vi "Stop Instruments.vi"(8 "Error In":errorcluster, 11 "reference in":refnum<class "Measure and Stimulus Subsystems.lvclass">) -> (0 "Error Out":errorcluster, 3 "reference out":refnum<class "Measure and Stimulus Subsystems.lvclass">)   [LabVIEW 2023, in "HAL GOOP4.lvlib" / "Measure and Stimulus Subsystems.lvclass"]
uses:
  Measure and Stimulus Subsystems.lvclass
  Measure and Stimulus Subsystems.lvclass/Measure and Stimulus Subsystems.ctl
  Interfaces/IInstrument/IInstrument.lvclass
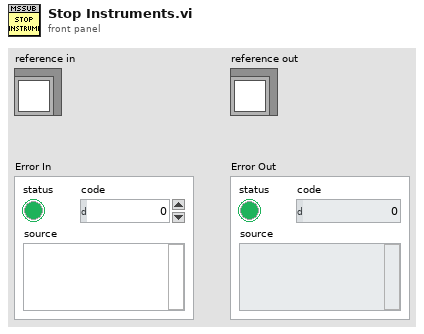
[diagram p1: front panel]
types:
  T1 = typedef "HAL GOOP4.lvlib/Measure and Stimulus Subsystems.lvclass/ObjectAttributes.ctl" = cluster{"Virt Instr":map{string, cluster{"IInstrument Base":refnum<class "IInstrument.lvclass">, "Channel":u8}}, "Physical Instr":map{string, cluster{"IInstrument Base":refnum<class "IInstrument.lvclass">, "Ref Count":u8}}}
  T2 = map{string, cluster{"IInstrument Base":refnum<class "IInstrument.lvclass">, "Ref Count":u8}}
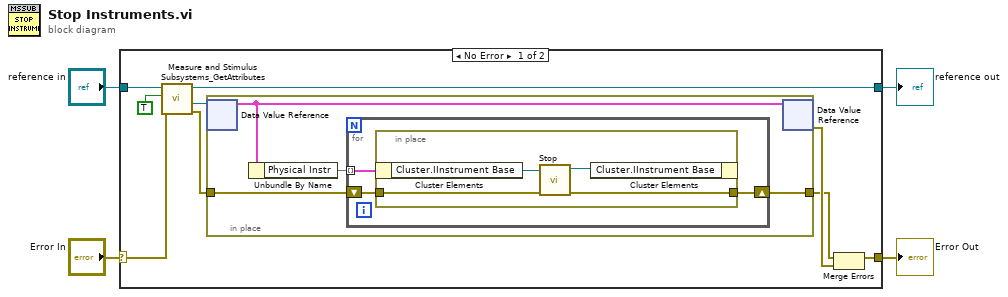
[diagram p0: block diagram]
diagram:
  n1 = case shown="No Error" "Error In" {
    selector: "Error In" -> [w12 w26]
    tunnel: [w9 w26] -> w3
    tunnel: [w10 w25] -> w1
    tunnel: "reference in" -> [w13 w25]
    frame No Error {
      n2 = call "Measure and Stimulus Subsystems_GetAttributes.vi"("Error In"=w12, "OnlyGetDvrReference(False)"=TRUE, "reference in"=w13) -> ("Error Out"=w6:errorcluster, "DataRef"=w8:refnum<data-value>, "reference out"=w10:refnum<class "Measure and Stimulus Subsystems.lvclass">)  [unwired: 5 in, 1 out]
      n3 = in-place {
        in-place-border: [w15] -> w5
        in-place-border: w6 -> [w14]
        n4 = in-place-dvr #1(w8) -> (w16:T1)  [unwired: 1 out]
        n5 = Unbundle By Name(w16) -> ("Physical Instr"=w17:T2)
        n6 = for {
          tunnel: w17 -> [w20] mode=indexing
          shift-right: [w18] -> w15
          shift-left: w14 -> [w19]
          n7 = in-place {
            in-place-border: w19 -> [w22]
            in-place-border: [w21] -> w18
            n8 = in-place-cluster #2(w20) -> ("Cluster.IInstrument Base"=w24:refnum<class "IInstrument.lvclass">)
            n9 = call-dynamic "Stop.vi"("Error In"=w22, "object in"=w24) -> ("Error Out"=w21:errorcluster, "object out"=w23:refnum<class "IInstrument.lvclass">)  [unwired: 8 in]
            n10 = in-place-cluster #2("Cluster.IInstrument Base"=w23) -> ()  [unwired: 1 out]
          }
        }
        n11 = in-place-dvr #1(w16) -> (w11:errorcluster)  [unwired: 1 out]
      }
      n12 = Merge Errors(w5, w11) -> (w9:errorcluster)
    }
    frame Error {
    }
  }
  "Error Out" <- w3
  "reference out" <- w1
